vi "Sets and Query the Reference Value for the Relative Function.vi"(5 "Enable to Query":bool=TRUE, 7 "Enable to Sets":bool=TRUE, 8 "error in":errorcluster, 10 "Reference Value":dbl format="%#.6g", 11 "VISA resource name":refnum<visa-resource-name>) -> (0 "error out":errorcluster, 2 "Return the Reference Value":string, 3 "VISA resource name out":refnum<visa-resource-name>)   [LabVIEW 2011, in "DMM4.lvlib"]
uses:
  <instrlib>/DMM4/DMM4.lvlib
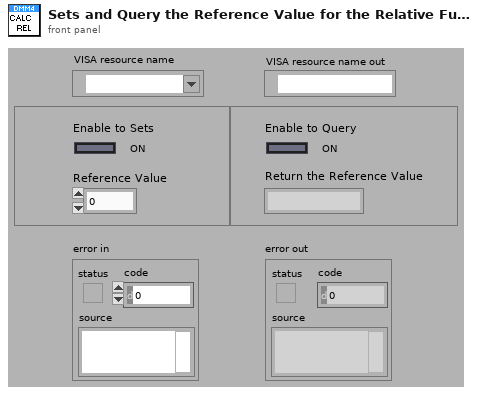
[diagram p1: front panel]
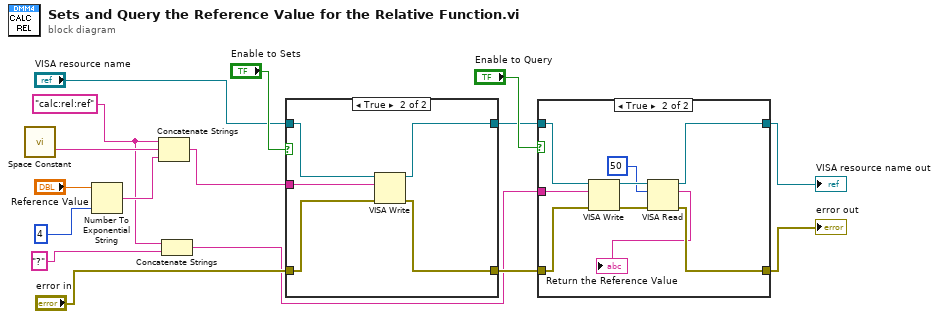
[diagram p0: block diagram]
diagram:
  w12 = "calc:rel:ref"
  n1 = call <vilib>:"Space Constant.vi"() -> ("String"=w14:string)
  n2 = Number To Exponential String(number="Reference Value", precision (6)=i16 4) -> (E-format string=w13:string)  [unwired: 2 in]
  n3 = Concatenate Strings(w12, w14, w13) -> (w7:string)
  n4 = Concatenate Strings(w12, "?") -> (w3:string)
  n5 = case shown="True" "Enable to Sets" {
    tunnel: "VISA resource name" -> [w18 w23]
    tunnel: "error in" -> [w17 w22]
    tunnel: [w18 w21] -> w5
    tunnel: [w17 w20] -> w4
    tunnel: w7 -> [_ w19]
    frame False {
    }
    frame True {
      n6 = VISA Write(VISA resource name=w23, write buffer=w19, error in (no error)=w22) -> (VISA resource name out=w21:refnum<visa-resource-name>, error out=w20:errorcluster)  [unwired: 1 out]
    }
  }
  n7 = case shown="True" "Enable to Query" {
    tunnel: w5 -> [w25 w31]
    tunnel: w4 -> [w24 w30]
    tunnel: [w25 w28] -> w2
    tunnel: [w24 w27] -> w1
    tunnel: w3 -> [_ w29]
    frame False {
    }
    frame True {
      n8 = VISA Write(VISA resource name=w31, write buffer=w29, error in (no error)=w30) -> (VISA resource name out=w33:refnum<visa-resource-name>, error out=w34:errorcluster)  [unwired: 1 out]
      n9 = VISA Read(VISA resource name=w33, byte count=u32 50, error in (no error)=w34) -> (VISA resource name out=w28:refnum<visa-resource-name>, read buffer=→"Return the Reference Value":string, error out=w27:errorcluster)  [unwired: 1 out]
    }
  }
  "VISA resource name out" <- w2
  "error out" <- w1
